vi "test Alignment.vi"(8 "error in (no error)":errorcluster, 11 "TestCase in":refnum<class "Buffers Tests.lvclass">=refnum) -> (0 "error out":errorcluster, 3 "TestCase out":refnum<class "Buffers Tests.lvclass">)   [LabVIEW 2021, in "Buffers Tests.lvclass"]
uses:
  Buffers Tests.lvclass
  Classes/Buffers/Buffers.lvclass
  Classes/Buffer/Buffer.lvclass
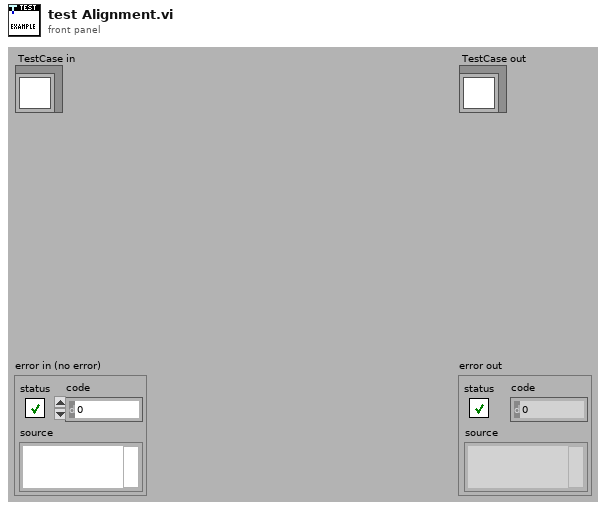
[diagram p1: front panel]
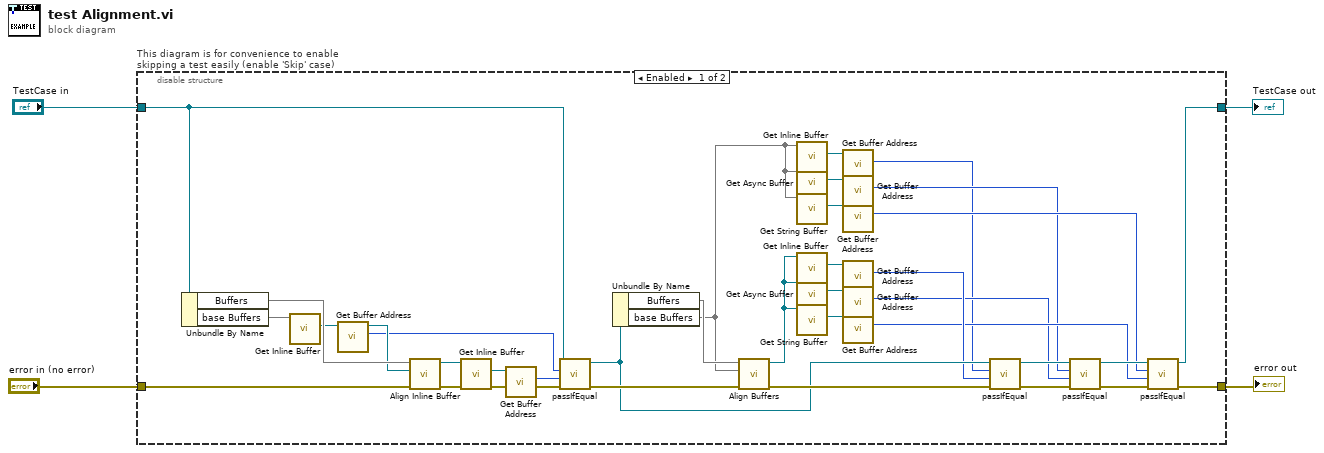
[diagram p0: block diagram]
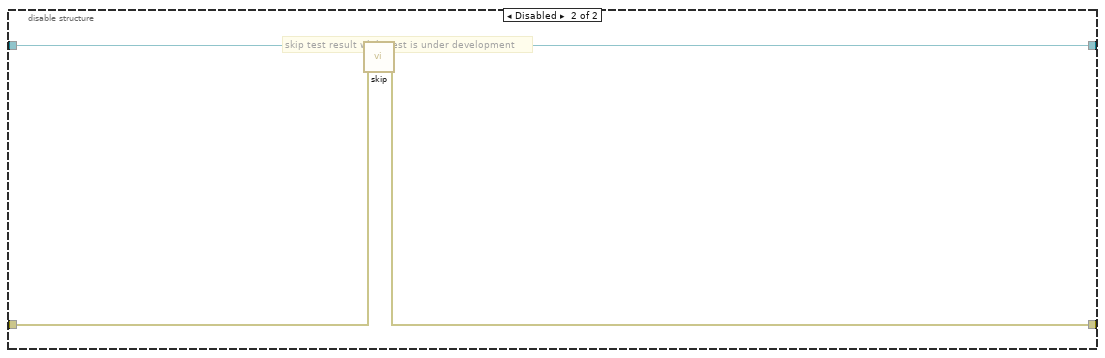
[diagram p2: hidden frame]
diagram:
  n1 = disable-structure "This diagram is for convenience to enable skipping a test easily (enable 'Skip' case)" shown="Enabled" {
    disable-tunnel: "TestCase in" -> [w37 w43]
    disable-tunnel: [w19 w41] -> w1
    disable-tunnel: [w20 w42] -> w3
    disable-tunnel: "error in (no error)" -> [w35 w40]
    frame Enabled {
      n2 = Unbundle By Name(w37) -> ("Buffers"=w36, "base Buffers"=w18)
      n3 = call "Get Inline Buffer.vi"("Buffers in"=w18) -> ("Inline Buffer"=w17:refnum<class "Buffer.lvclass">)  [unwired: 9 in, 1 out]
      n4 = call "Get Buffer Address.vi"("Buffer in"=w17) -> ("buffer address"=w29:u64, "Buffer out"=w30:refnum<class "Buffer.lvclass">)  [unwired: 9 in]
      n5 = call "Align Inline Buffer.vi"("error in (no error)"=w35, "base Inline Buffer"=w30, "Buffers in"=w36) -> ("error out"=w32:errorcluster, "Buffers out"=w34:refnum<class "Buffers.lvclass">)  [unwired: 7 in]
      n6 = call "Get Inline Buffer.vi"("Buffers in"=w34) -> ("Inline Buffer"=w33:refnum<class "Buffer.lvclass">)  [unwired: 9 in, 1 out]
      n7 = call "Get Buffer Address.vi"("Buffer in"=w33) -> ("buffer address"=w31:u64)  [unwired: 9 in, 1 out]
      n8 = call-dynamic "passIfEqual.vi"("error in (no error)"=w32, "y"=w31, "x"=w29, "TestCase in"=w37) -> ("error out"=w28:errorcluster, "TestCase out"=w11:refnum<class "Buffers Tests.lvclass">)  [unwired: 6 in]
      n9 = Unbundle By Name(w11) -> ("Buffers"=w21, "base Buffers"=w15)
      n10 = call "Align Buffers.vi"("error in (no error)"=w28, "base Buffers"=w15, "Buffers in"=w21) -> ("error out"=w12:errorcluster, "Buffers out"=w16:refnum<class "Buffers.lvclass">)  [unwired: 7 in]
      n11 = call "Get Inline Buffer.vi"("Buffers in"=w15) -> ("Inline Buffer"=w27:refnum<class "Buffer.lvclass">)  [unwired: 9 in, 1 out]
      n12 = call "Get Async Buffer.vi"("Buffers in"=w15) -> ("Async Buffer"=w25:refnum<class "Buffer.lvclass">)  [unwired: 9 in, 1 out]
      n13 = call "Get String Buffer.vi"("Buffers in"=w15) -> ("String Buffer"=w26:refnum<class "Buffer.lvclass">)  [unwired: 9 in, 1 out]
      n14 = call "Get Inline Buffer.vi"("Buffers in"=w16) -> ("Inline Buffer"=w24:refnum<class "Buffer.lvclass">)  [unwired: 9 in, 1 out]
      n15 = call "Get Async Buffer.vi"("Buffers in"=w16) -> ("Async Buffer"=w22:refnum<class "Buffer.lvclass">)  [unwired: 9 in, 1 out]
      n16 = call "Get String Buffer.vi"("Buffers in"=w16) -> ("String Buffer"=w23:refnum<class "Buffer.lvclass">)  [unwired: 9 in, 1 out]
      n17 = call "Get Buffer Address.vi"("Buffer in"=w27) -> ("buffer address"=w5:u64)  [unwired: 9 in, 1 out]
      n18 = call "Get Buffer Address.vi"("Buffer in"=w25) -> ("buffer address"=w6:u64)  [unwired: 9 in, 1 out]
      n19 = call "Get Buffer Address.vi"("Buffer in"=w26) -> ("buffer address"=w9:u64)  [unwired: 9 in, 1 out]
      n20 = call "Get Buffer Address.vi"("Buffer in"=w24) -> ("buffer address"=w10:u64)  [unwired: 9 in, 1 out]
      n21 = call "Get Buffer Address.vi"("Buffer in"=w22) -> ("buffer address"=w7:u64)  [unwired: 9 in, 1 out]
      n22 = call "Get Buffer Address.vi"("Buffer in"=w23) -> ("buffer address"=w8:u64)  [unwired: 9 in, 1 out]
      n23 = call-dynamic "passIfEqual.vi"("error in (no error)"=w12, "y"=w10, "x"=w5, "TestCase in"=w11) -> ("error out"=w13:errorcluster, "TestCase out"=w38:refnum<class "Buffers Tests.lvclass">)  [unwired: 6 in]
      n24 = call-dynamic "passIfEqual.vi"("error in (no error)"=w13, "y"=w7, "x"=w6, "TestCase in"=w38) -> ("error out"=w14:errorcluster, "TestCase out"=w39:refnum<class "Buffers Tests.lvclass">)  [unwired: 6 in]
      n25 = call-dynamic "passIfEqual.vi"("error in (no error)"=w14, "y"=w8, "x"=w9, "TestCase in"=w39) -> ("error out"=w20:errorcluster, "TestCase out"=w19:refnum<class "Buffers Tests.lvclass">)  [unwired: 6 in]
    }
    frame Disabled {
      # "skip test result while test is under development"
      n26 = call <vilib>:"skip.vi"("error in (no error)"=w40, "TestCase in"=w43) -> ("error out"=w42:errorcluster, "TestCase out"=w41:refnum<class "Buffers Tests.lvclass">)  [unwired: 8 in]
    }
  }
  "error out" <- w3
  "TestCase out" <- w1
